vi "Variable_Open Compilation.vi"(0 "scripts manager in":refnum<class "scripts manager.lvclass">, 5 "function in":refnum<class "functionbase.lvclass">, 7 "Variables Name":string[](array[string]), 9 "Variables Value":string[](array[string]), 11 "error in (no error)":errorcluster) -> (4 "scripts manager out":refnum<class "scripts manager.lvclass">, 6 "function":refnum<class "functionbase.lvclass">, 8 "Compilation passed?":bool, 15 "error out":errorcluster)   [LabVIEW 2019, in "LSL.lvlib" / "scripts manager.lvclass"]
uses:
  scripts manager.lvclass
  functions/functionsbase/functionbase.lvclass
  functions/functionsbase/functionbase.lvclass/functionbase.ctl
  common/variable utils/Valuetype.ctl
  functions/functionsbase/properties/Read Line#.vi
  functions/functionsbase/properties/Read Indent#.vi
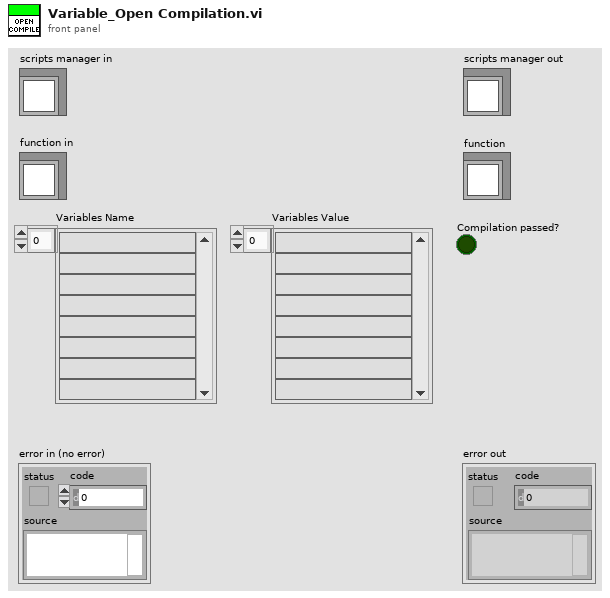
[diagram p1: front panel]
types:
  T1 = typedef "Valuetype.ctl" = enum16{"Value", "Variable", "Function"}
  T2 = typedef "Datatype.ctl" = enum16{"Null", "Numeric", "String", "Bool", "Numeric 1D", "String 1D", "Bool 1D", "Numeric 2D", "String 2D", "Bool 2D", "Variant"}
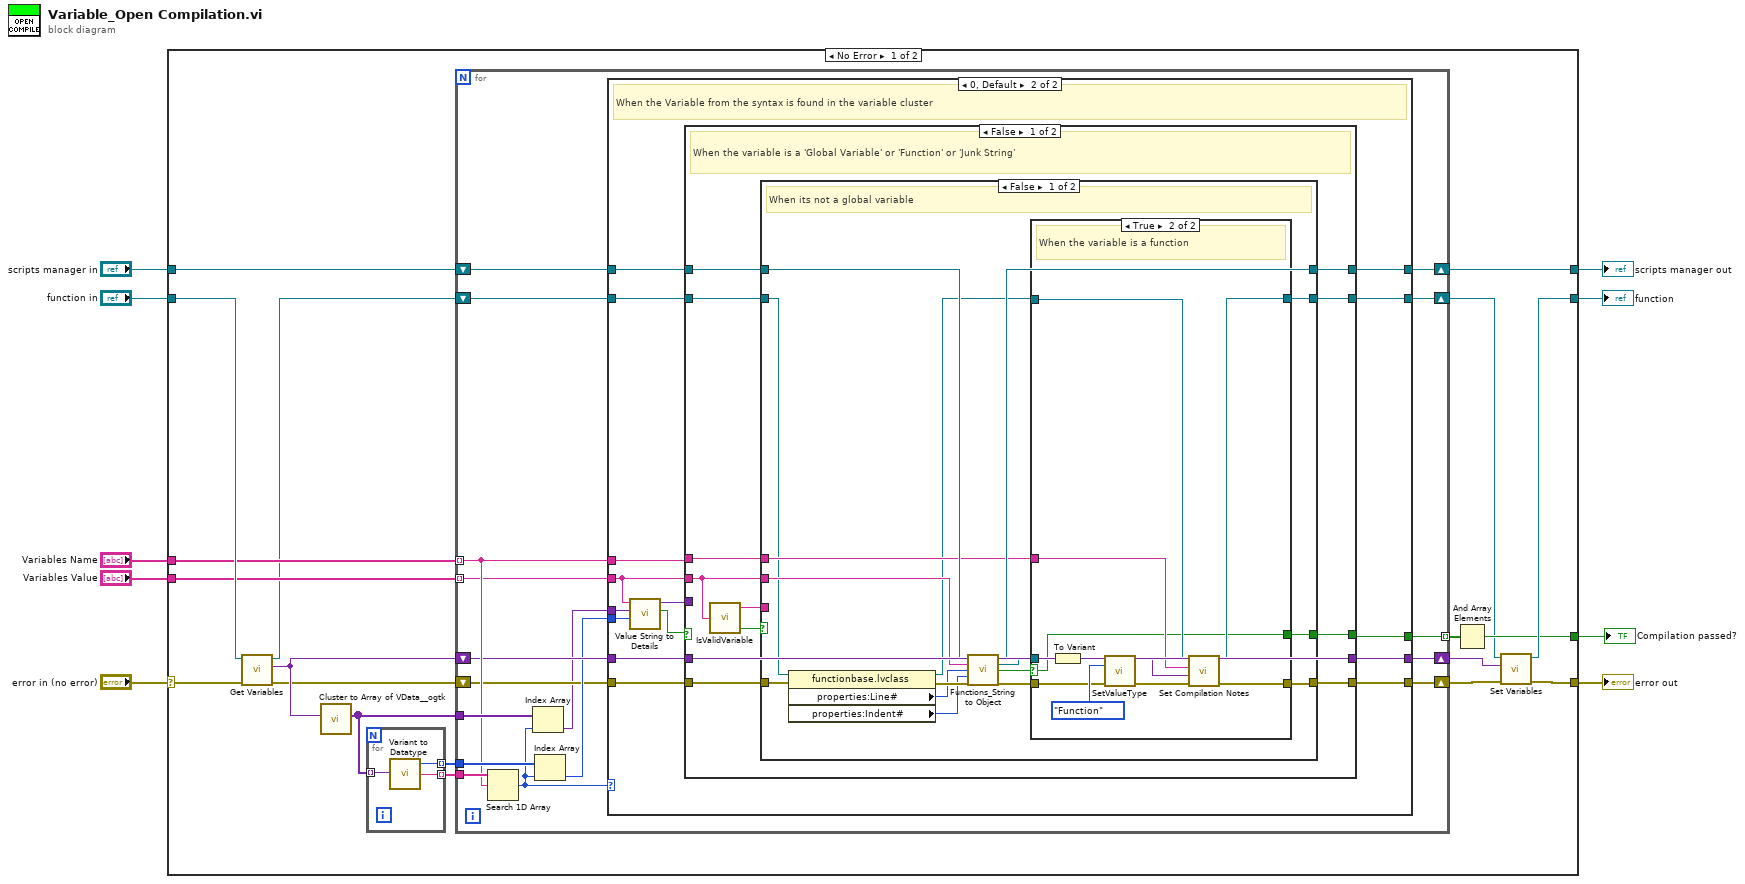
[diagram p0: block diagram]
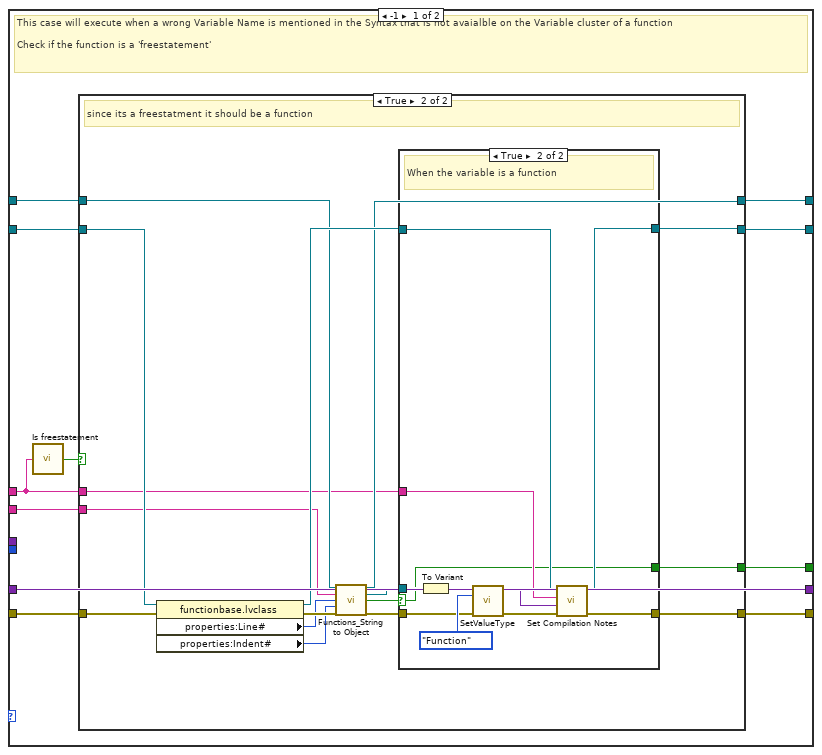
[diagram p2: hidden frame]
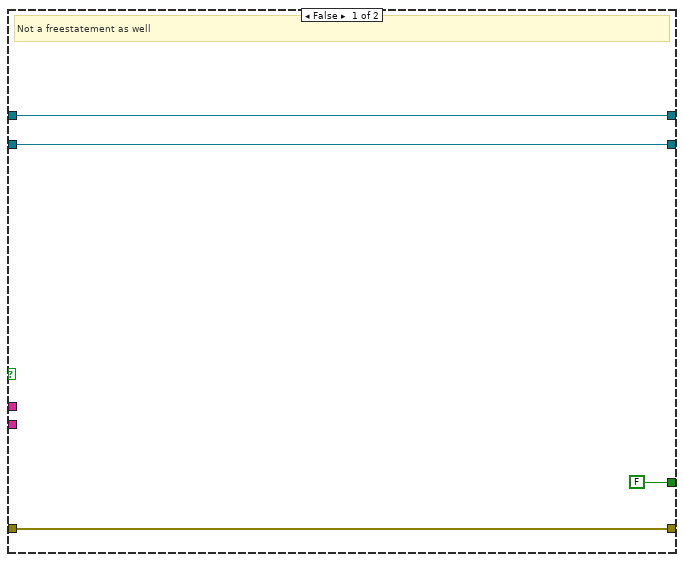
[diagram p3: hidden frame]
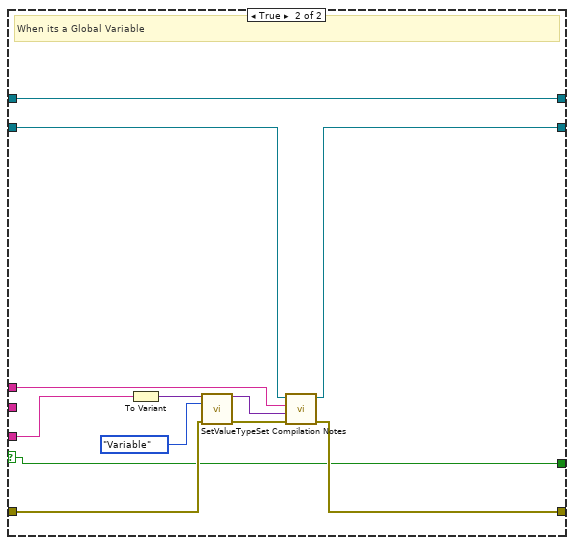
[diagram p6: hidden frame]
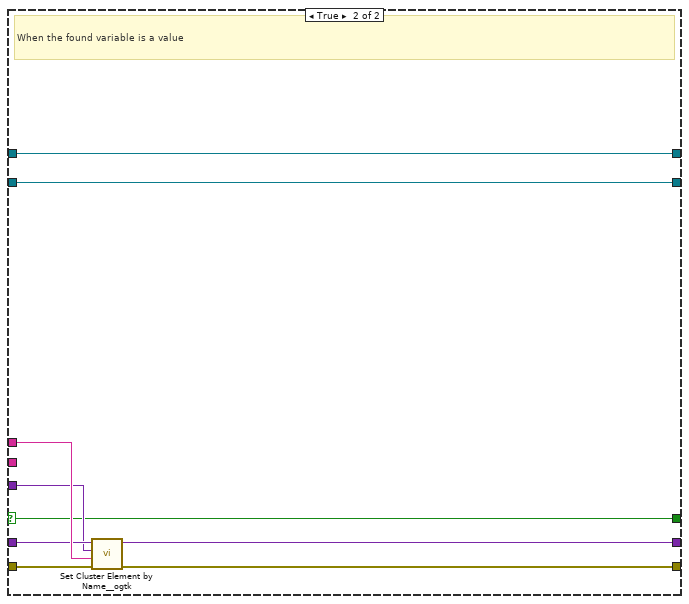
[diagram p7: hidden frame]
diagram:
  n1 = case shown="No Error" "error in (no error)" {
    selector: "error in (no error)" -> [w27 w173]
    tunnel: [w25 w173] -> w8
    tunnel: [w16 w172] -> w6
    tunnel: "scripts manager in" -> [w17 w172]
    tunnel: "function in" -> [w28 _]
    tunnel: [w26 _] -> w4
    tunnel: "Variables Name" -> [w21 _]
    tunnel: "Variables Value" -> [w20 _]
    tunnel: [w12 _] -> w1
    frame No Error {
      n2 = call-dynamic "Get Variables.vi"("error in (no error)"=w27, "functionbase in"=w28) -> ("error out"=w18:errorcluster, "Variables"=w19:variant, "functionbase out"=w11:refnum<class "functionbase.lvclass">)  [unwired: 7 in]
      n3 = call <userlib>:"Cluster to Array of VData__ogtk.vi"("Cluster"=w19) -> ("Array of VData"=w24:variant[])  [unwired: 9 in, 1 out]
      n4 = for {
        tunnel: w24 -> [w171] mode=indexing
        tunnel: [w170] -> w23 mode=indexing
        tunnel: [w169] -> w22 mode=indexing
        n5 = call "Variant to Datatype.vi"("Variant"=w171) -> ("Name"=w169:string, "Datatype"=w170:T2)  [unwired: 2 in, 1 out]
      }
      n6 = for {
        shift-right: [w41] -> w14
        shift-left: w19 -> [w40]
        shift-right: [w39] -> w15
        shift-left: w18 -> [w36]
        tunnel: w24 -> [w43]
        tunnel: w23 -> [w44]
        tunnel: w22 -> [w45]
        tunnel: w21 -> [w42] mode=indexing
        tunnel: w20 -> [w37] mode=indexing
        shift-right: [w29] -> w16
        shift-left: w17 -> [w30]
        tunnel: [w35] -> w13 mode=indexing
        shift-right: [w32] -> w10
        shift-left: w11 -> [w31]
        n7 = Search 1D Array(1D array=w45, element=w42) -> (index of element=w34:i32)  [unwired: 1 in]
        n8 = Index Array(array=w43, index=w34) -> (element=w33:variant)
        n9 = Index Array(array=w44, index=w34) -> (element=w38:T2)
        n10 = case shown="0, Default" w34 {
          tunnel: w42 -> [w47 w105]
          tunnel: [w56 w104] -> w41
          tunnel: w40 -> [w56 w103]
          tunnel: [w49 w102] -> w39
          tunnel: w38 -> [_ w101]
          tunnel: w37 -> [w46 w95]
          tunnel: w36 -> [w48 w100]
          tunnel: [w54 w97] -> w35
          tunnel: w33 -> [_ w96]
          tunnel: [w50 w94] -> w32
          tunnel: w31 -> [w51 w93]
          tunnel: w30 -> [w52 w92]
          tunnel: [w53 w91] -> w29
          frame -1 {
            # "This case will execute when a wrong Variable Name is mentioned in the Syntax that is not avaialble on the Variable cluster of a function\n\nCheck if the function is a 'freestatement'"
            n11 = call "Is freestatement.vi"("Variable Name"=w47) -> ("freestatement?"=w55:bool)
            n12 = case shown="True" w55 {
              tunnel: [FALSE w63] -> w54
              tunnel: [w59 w67] -> w53
              tunnel: w52 -> [w59 w69]
              tunnel: w51 -> [w58 w68]
              tunnel: [w58 w66] -> w50
              tunnel: [w57 w64] -> w49
              tunnel: w48 -> [w57 w65]
              tunnel: w47 -> [_ w62]
              tunnel: w46 -> [_ w61]
              frame False {
                # "Not a freestatement as well"
              }
              frame True {
                # "since its a freestatment it should be a function"
                n13 = property class="functionbase.lvclass"(reference=w68, error in=w65) -> (reference out=w70:refnum<class "functionbase.lvclass">, error out=w73:errorcluster, "properties:Line#"=w72:i64, "properties:Indent#"=w71:i64)
                n14 = call-dynamic "Functions_String to Object.vi"("scripts manager in"=w69, "Functions"=w61, "Line#"=w72, "Indent#"=w71, "error in (no error)"=w73) -> ("scripts manager out"=w67:refnum<class "scripts manager.lvclass">, "function obj"=w76:refnum<class "functionbase.lvclass">, "function created"=w74:bool, "error out"=w75:errorcluster)  [unwired: 7 in]
                n15 = case shown="True" w74 {
                  selector: w74 -> [w77 w80]
                  tunnel: w76 -> [_ w86]
                  tunnel: w75 -> [w78 w85]
                  tunnel: w62 -> [_ w84]
                  tunnel: w70 -> [w79 w83]
                  tunnel: [w79 w82] -> w66
                  tunnel: [w78 w81] -> w64
                  tunnel: [w77 w80] -> w63
                  frame False {
                    # "When its not a function"
                  }
                  frame True {
                    # "When the variable is a function"
                    n16 = To Variant(anything=w86) -> (Variant=w89:variant)
                    n17 = call "SetValueType.vi"("variant"=w89, "valuetype"=Valuetype."Function", "error in"=w85) -> ("variant out"=w88:variant, "error out"=w87:errorcluster)  [unwired: 11 in]
                    n18 = call "Set Compilation Notes.vi"("error in (no error)"=w87, "Notes"=w88, "note key"=w84, "functionbase in"=w83) -> ("error out"=w81:errorcluster, "functionbase out"=w82:refnum<class "functionbase.lvclass">)  [unwired: 6 in]
                  }
                }
              }
            }
          }
          frame 0, Default {
            # "When the Variable from the syntax is found in the variable cluster"
            n19 = call "Value String to Details.vi"("Datatype"=w101, "Default"=w96, "Value String"=w95) -> ("Identified?"=w98:bool, "Value Variant"=w99:variant)  [unwired: 7 in]
            n20 = case shown="False" w98 {
              selector: w98 -> [_ w162]
              tunnel: w105 -> [w115 w168]
              tunnel: [w117 w167] -> w104
              tunnel: w103 -> [w117 w166]
              tunnel: [w114 w165] -> w102
              tunnel: w100 -> [w112 w164]
              tunnel: w99 -> [_ w163]
              tunnel: [w106 w162] -> w97
              tunnel: w95 -> [w107 _]
              tunnel: [w111 w161] -> w94
              tunnel: w93 -> [w116 w161]
              tunnel: w92 -> [w109 w160]
              tunnel: [w108 w160] -> w91
              frame False {
                # "When the variable is a 'Global Variable' or 'Function' or 'Junk String'"
                n21 = call "IsValidVariable.vi"("Value String in"=w107) -> ("IsVariable"=w110:bool, "Variable Name"=w113:string)  [unwired: 3 in]
                n22 = case shown="False" w110 {
                  selector: w110 -> [_ w148]
                  tunnel: w116 -> [w119 w159]
                  tunnel: w115 -> [w128 w158]
                  tunnel: [w126 w157] -> w114
                  tunnel: w113 -> [_ w155]
                  tunnel: w112 -> [w123 w151]
                  tunnel: [w127 w150] -> w111
                  tunnel: w109 -> [w133 w149]
                  tunnel: [w131 w149] -> w108
                  tunnel: w107 -> [w132 _]
                  tunnel: [w124 w148] -> w106
                  frame False {
                    # "When its not a global variable"
                    n23 = property class="functionbase.lvclass"(reference=w119, error in=w123) -> (reference out=w118:refnum<class "functionbase.lvclass">, error out=w122:errorcluster, "properties:Line#"=w121:i64, "properties:Indent#"=w120:i64)
                    n24 = call-dynamic "Functions_String to Object.vi"("scripts manager in"=w133, "Functions"=w132, "Line#"=w121, "Indent#"=w120, "error in (no error)"=w122) -> ("scripts manager out"=w131:refnum<class "scripts manager.lvclass">, "function obj"=w130:refnum<class "functionbase.lvclass">, "function created"=w125:bool, "error out"=w129:errorcluster)  [unwired: 7 in]
                    n25 = case shown="True" w125 {
                      selector: w125 -> [w134 w137]
                      tunnel: w130 -> [_ w143]
                      tunnel: w129 -> [w135 w142]
                      tunnel: w128 -> [_ w141]
                      tunnel: w118 -> [w136 w140]
                      tunnel: [w136 w139] -> w127
                      tunnel: [w135 w138] -> w126
                      tunnel: [w134 w137] -> w124
                      frame False {
                        # "When its not a function"
                      }
                      frame True {
                        # "When the variable is a function"
                        n26 = To Variant(anything=w143) -> (Variant=w146:variant)
                        n27 = call "SetValueType.vi"("variant"=w146, "valuetype"=Valuetype."Function", "error in"=w142) -> ("variant out"=w145:variant, "error out"=w144:errorcluster)  [unwired: 11 in]
                        n28 = call "Set Compilation Notes.vi"("error in (no error)"=w144, "Notes"=w145, "note key"=w141, "functionbase in"=w140) -> ("error out"=w138:errorcluster, "functionbase out"=w139:refnum<class "functionbase.lvclass">)  [unwired: 6 in]
                      }
                    }
                  }
                  frame True {
                    # "When its a Global Variable"
                    n29 = To Variant(anything=w155) -> (Variant=w154:variant)
                    n30 = call "SetValueType.vi"("variant"=w154, "valuetype"=Valuetype."Variable", "error in"=w151) -> ("variant out"=w153:variant, "error out"=w152:errorcluster)  [unwired: 11 in]
                    n31 = call "Set Compilation Notes.vi"("error in (no error)"=w152, "Notes"=w153, "note key"=w158, "functionbase in"=w159) -> ("error out"=w157:errorcluster, "functionbase out"=w150:refnum<class "functionbase.lvclass">)  [unwired: 6 in]
                  }
                }
              }
              frame True {
                # "When the found variable is a value"
                n32 = call <userlib>:"Set Cluster Element by Name__ogtk.vi"("error in (no error)"=w164, "Element Name (\"\": New Element Data Name)"=w168, "New Element Value"=w163, "Cluster"=w166) -> ("error out"=w165:errorcluster, "VCluster out"=w167:variant)  [unwired: 5 in, 1 out]
              }
            }
          }
        }
      }
      n33 = And Array Elements(Boolean array=w13) -> (logical AND=w12:bool)
      n34 = call-dynamic "Set Variables.vi"("error in (no error)"=w15, "Variables"=w14, "functionbase in"=w10) -> ("error out"=w25:errorcluster, "functionbase out"=w26:refnum<class "functionbase.lvclass">)  [unwired: 7 in]
    }
    frame Error {
    }
  }
  "error out" <- w8
  "scripts manager out" <- w6
  "function" <- w4
  "Compilation passed?" <- w1
